vi "8bit sync-Create IMAQ image refs.vi"() -> (3 "8-bit Image refs cluster":T1)   [LabVIEW 2017]
uses:
  Typedefs/8bit sync-IMAQ image refs.ctl
  <vilib>/vision/Image Controls.llb/IMAQ Image.ctl
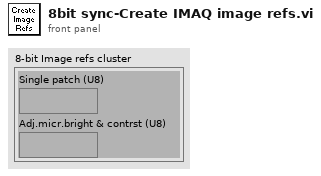
[diagram p1: front panel]
types:
  T1 = typedef "8bit sync-IMAQ image refs.ctl" = cluster{"Single patch (U8)":T2, "Adj.micr.bright & contrst (U8)":T2}
  T2 = typedef "IMAQ Image.ctl" = refnum<image>
  T3 = typedef "Image Type" = u32
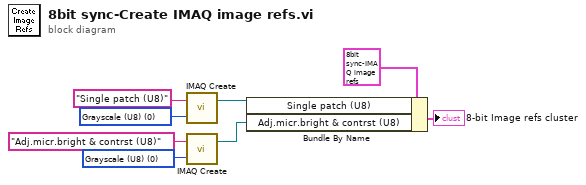
[diagram p0: block diagram]
diagram:
  w4 = T3 0 items=["Grayscale (U8)", "Grayscale (I16)", "Grayscale (SGL)", "Complex (CSG)", "RGB (U32)", "HSL (U32)", "RGB (U64)", "Grayscale (U16)"] ("Image Type")
  w7 = T3 0 items=["Grayscale (U8)", "Grayscale (I16)", "Grayscale (SGL)", "Complex (CSG)", "RGB (U32)", "HSL (U32)", "RGB (U64)", "Grayscale (U16)"] ("Image Type")
  n1 = call "IMAQ Create"("Image Name"="Single patch (U8)", "Image Type"=w7) -> ("New Image"=w8:T2)  [unwired: 2 in, 2 out]
  n2 = call "IMAQ Create"("Image Name"="Adj.micr.bright & contrst (U8)", "Image Type"=w4) -> ("New Image"=w2:T2)  [unwired: 3 in, 1 out]
  n3 = Bundle By Name(cluster=T1 {"Single patch (U8)"=refnum, "Adj.micr.bright & contrst (U8)"=refnum} ("8-bit Image refs cluster"), "Single patch (U8)"=w8, "Adj.micr.bright & contrst (U8)"=w2) -> (→"8-bit Image refs cluster":T1)
